vi "DELETE.vi"(6 "timeout":i32=10000, 7 "output file":path, 8 "error in":errorcluster, 10 "url":string, 11 "http-client in":refnum<class "http-client.lvclass">) -> (0 "error out":errorcluster, 1 "body":string, 2 "headers":string, 3 "http-client out":refnum<class "http-client.lvclass">, 4 "status code":u16)   [LabVIEW 2025, in "http-client.lvclass"]
uses:
  http-client.lvclass
  REST Client/REST Client.lvclass
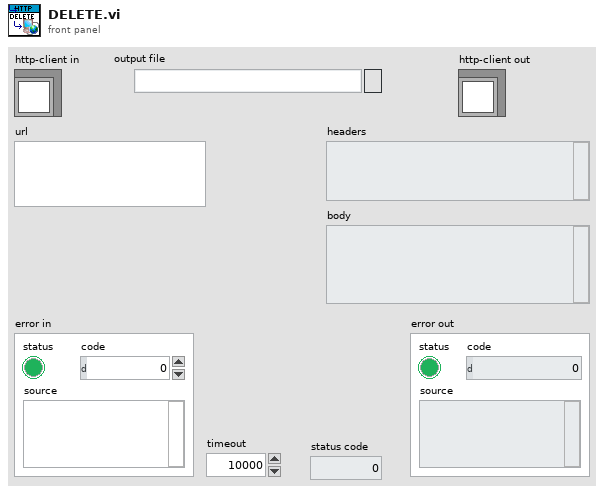
[diagram p1: front panel]
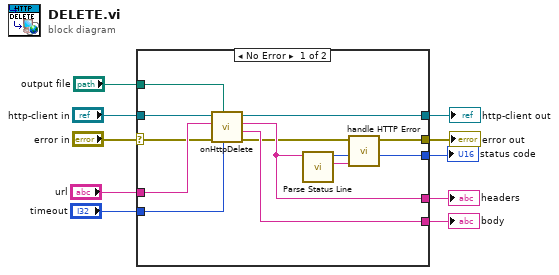
[diagram p0: block diagram]
diagram:
  n1 = case shown="No Error" "error in" {
    selector: "error in" -> [w20 w25]
    tunnel: [w14 w25] -> w9
    tunnel: [w19 w24] -> w7
    tunnel: "http-client in" -> [w22 w24]
    tunnel: [w16 _] -> w6
    tunnel: "url" -> [w21 _]
    tunnel: "timeout" -> [w17 _]
    tunnel: "output file" -> [w23 _]
    tunnel: [w18 _] -> w2
    tunnel: [w12 _] -> w1
    frame No Error {
      n2 = call-dynamic "onHttpDelete.vi"("timeout"=w17, "output file"=w23, "error in"=w20, "url"=w21, "http-method in"=w22) -> ("error out"=w15:errorcluster, "body"=w18:string, "headers"=w16:string, "http-method out"=w19:refnum<class "http-client.lvclass">)  [unwired: 3 in]
      n3 = call "Parse Status Line.vi"("Headers w/ status line"=w16) -> ("Status String"=w11:string, "status code"=w13:u16)  [unwired: 6 in, 3 out]
      n4 = call "handle HTTP Error.vi"("Status String"=w11, "status code"=w13, "error in (no error)"=w15) -> ("status code dup"=w12:u16, "error out"=w14:errorcluster)  [unwired: 7 in]
    }
    frame Error {
    }
  }
  "error out" <- w9
  "http-client out" <- w7
  "headers" <- w6
  "body" <- w2
  "status code" <- w1
